vi "gaussfit_subvi.vi"(11 "Refnum in":T1) -> (3 "Refnum out":T1)   [LabVIEW 2020]
uses:
  <vilib>/vision/Image Controls.llb/IMAQ Image.ctl
panel:
  out "Waveform Graph":i32[](graph)
  out "output array":i32[](array[numeric])
  out "size(s) 2":i32[](array[numeric])
  out "Image Pixels (U8) 2":u8[](array[numeric])
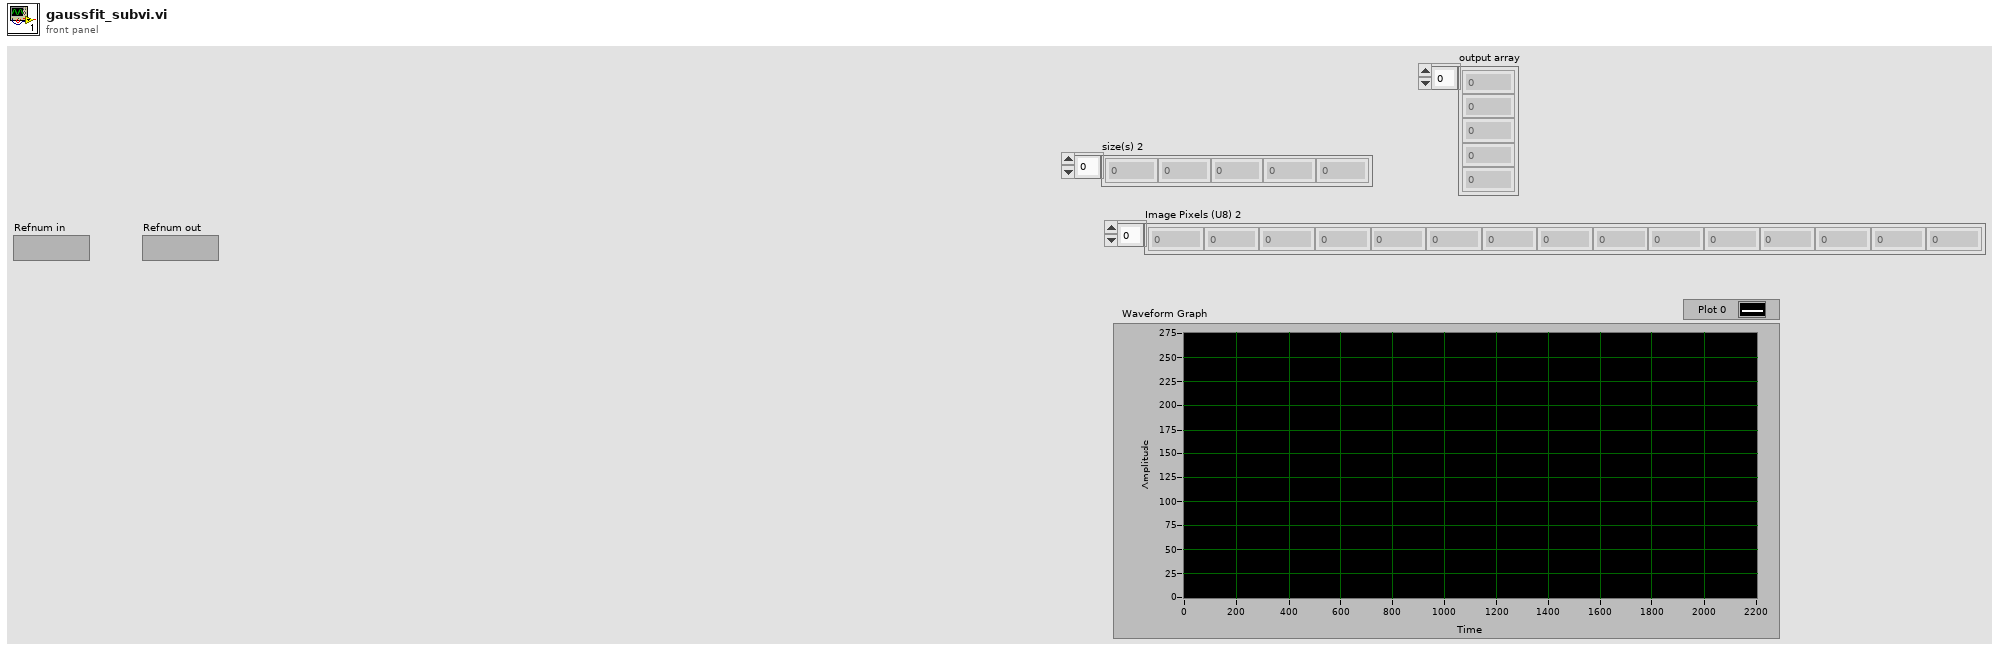
[diagram p1: front panel]
types:
  T1 = typedef "IMAQ Image.ctl" = refnum<image>
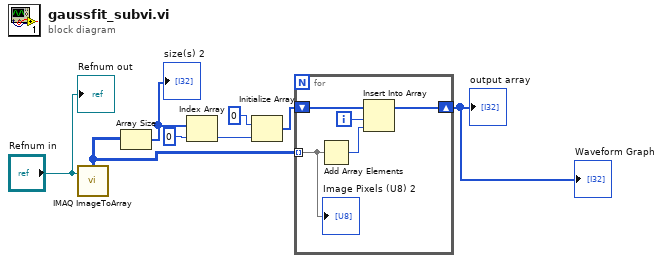
[diagram p0: block diagram]
diagram:
  n1 = call "IMAQ ImageToArray"("Image"="Refnum in") -> ("Image Pixels (U8)"=w7:u8[][])  [unwired: 3 in, 4 out]
  n2 = Array Size(array=w7) -> (size(s)=w6:i32[])
  "size(s) 2" <- w6
  n3 = Index Array(array=w6, index=0) -> (element=w4:i32)
  n4 = Initialize Array(0, w4) -> (w2:i32[])
  n5 = for {
    tunnel: w7 -> [w13] mode=indexing
    shift-right: [w10] -> w1
    shift-left: w2 -> [w12]
    i -> [w9]
    n6 = Add Array Elements(numeric array=w13) -> (sum=w11:u8)
    n7 = Insert Into Array(array=w12, index=w9, new element=w11) -> (w10:i32[])
    "Image Pixels (U8) 2" <- w13
  }
  "output array" <- w1
  "Waveform Graph" <- w1
  "Refnum out" <- "Refnum in"
